vi "Read Stop When Parent Stopped.vi"(11 "Core Actor in":refnum<class "Core Actor.lvclass">) -> (2 "Stop When Parent Stopped":bool)   [LabVIEW 2025, in "jettl.lvlib" / "Core Actor.lvlib" / "Core Actor.lvclass"]
uses:
  Core Actor.lvclass
  Core Actor.lvclass/Core Actor.ctl
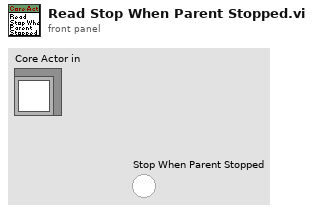
[diagram p1: front panel]
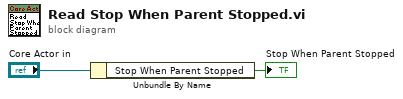
[diagram p0: block diagram]
diagram:
  n1 = Unbundle By Name("Core Actor in") -> ("Stop When Parent Stopped"=→"Stop When Parent Stopped":bool)
